vi "RandomNumber.vi"() -> (3 "Numeric":i32)   [LabVIEW 2022 SP3]
panel:
  # "Well Use a State machine style approch.\nWell make 4 buttons that represent the states\n\"00\" \"01\" \"10\" \"11\""
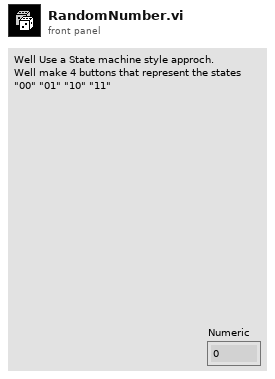
[diagram p1: front panel]
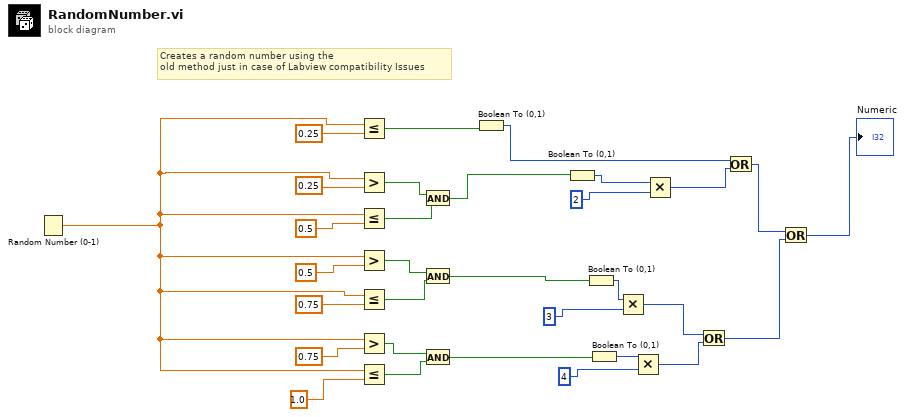
[diagram p0: block diagram]
diagram:
  # "Creates a random number using the \nold method just in case of Labview compatibility Issues"
  n1 = Random Number (0-1)() -> (number: 0 to 1=w25:dbl)
  n2 = Less Or Equal?(x=w25, y=0.25) -> (x <= y?=w14:bool)
  n3 = Greater?(x=w25, y=0.25) -> (0:w23:bool)
  n4 = Less Or Equal?(x=w25, y=0.5) -> (x <= y?=w22:bool)
  n5 = Greater?(x=w25, y=0.5) -> (0:w21:bool)
  n6 = Less Or Equal?(x=w25, y=0.75) -> (x <= y?=w20:bool)
  n7 = Greater?(x=w25, y=0.75) -> (0:w19:bool)
  n8 = Less Or Equal?(x=w25, y=1.0) -> (x <= y?=w18:bool)
  n9 = And(x=w23, y=w22) -> (x .and. y?=w15:bool)
  n10 = And(x=w21, y=w20) -> (x .and. y?=w16:bool)
  n11 = And(x=w19, y=w18) -> (x .and. y?=w17:bool)
  n12 = Boolean To (0,1)(Boolean=w14) -> (0, 1=w11:i16)
  n13 = Boolean To (0,1)(Boolean=w15) -> (0, 1=w12:i16)
  n14 = Boolean To (0,1)(Boolean=w16) -> (0, 1=w6:i16)
  n15 = Boolean To (0,1)(Boolean=w17) -> (0, 1=w7:i16)
  n16 = Multiply(x=w6, y=3) -> (x*y=w5:i32)
  n17 = Multiply(x=w7, y=4) -> (x*y=w4:i32)
  n18 = Multiply(x=w12, y=2) -> (x*y=w10:i32)
  n19 = Or(x=w5, y=w4) -> (x .or. y?=w2:i32)
  n20 = Or(x=w11, y=w10) -> (x .or. y?=w3:i32)
  n21 = Or(x=w3, y=w2) -> (x .or. y?=→"Numeric":i32)
